vi "Swerve Sensors Read.vi"(11 "Swerve Motor DevRef":T1) -> ()   [LabVIEW 2014]
uses:
  Swerve Sensors DevRef.ctl
  <vilib>/Rock Robotics/WPI/AnalogChannel/WPI_AnalogChannelDevRef.ctl
  <vilib>/Rock Robotics/SystemInterfaces/Typedef/FPGA_TypedefAnalogModule.ctl
  <vilib>/Rock Robotics/SystemInterfaces/AI/FPGA_AIChannel.ctl
  Global Variables/Sensor Data (Edited).vi
  Global Variables/Calibrations.vi
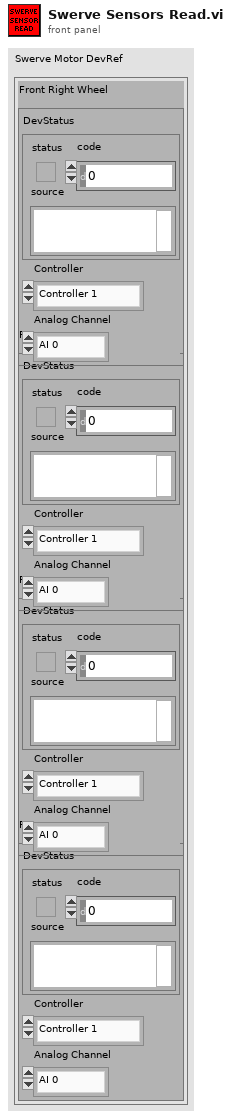
[diagram p1: front panel]
types:
  T1 = typedef "Swerve Sensors DevRef.ctl" = cluster{"Front Right Wheel":T2, "Front Left Wheel":T2, "Rear Right Wheel":T2, "Rear Left Wheel":T2}
  T2 = typedef "WPI_AnalogChannelDevRef.ctl" = cluster{"DevStatus":errorcluster, "Controller":T3, "Analog Channel":T4}
  T3 = typedef "FPGA_TypedefAnalogModule.ctl" = enum16{"Controller 1"}
  T4 = typedef "FPGA_AIChannel.ctl" = enum8{"AI 0", "AI 1", "AI 2", "AI 3", "AI MXP 0", "AI MXP 1", "AI MXP 2", "AI MXP 3", "Invalid"}
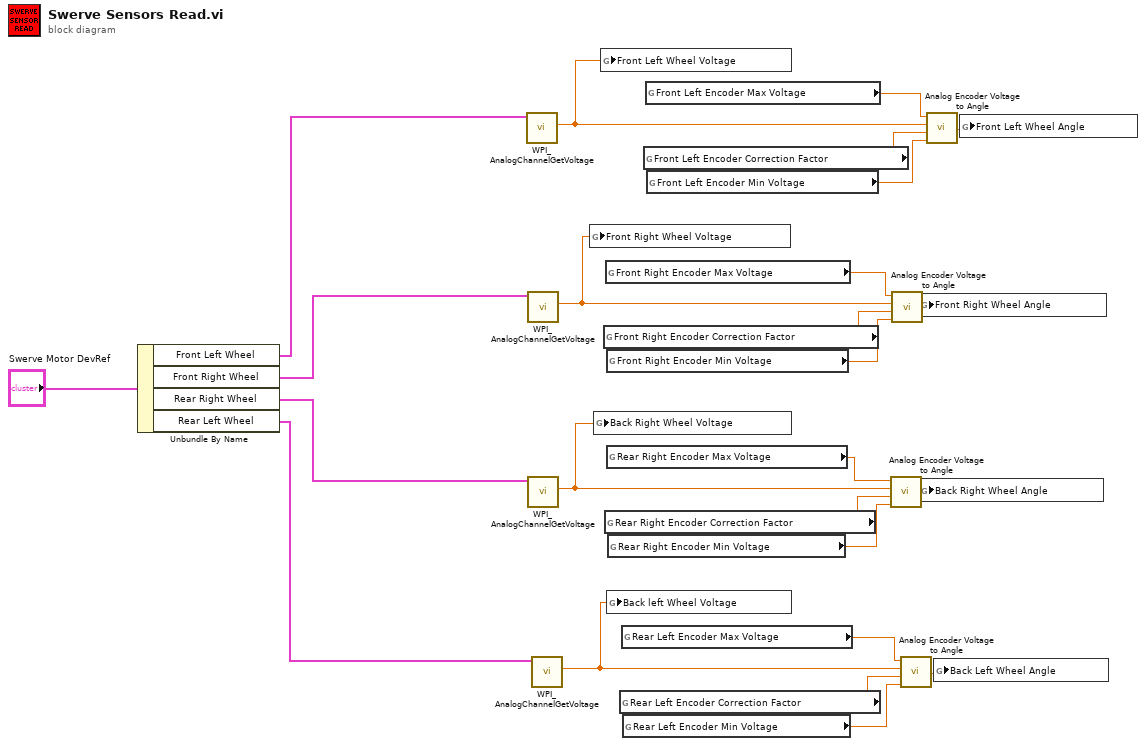
[diagram p0: block diagram]
diagram:
  n1 = Unbundle By Name("Swerve Motor DevRef") -> ("Front Left Wheel"=w24:T2, "Front Right Wheel"=w23:T2, "Rear Right Wheel"=w22:T2, "Rear Left Wheel"=w21:T2)
  n2 = call <vilib>:"WPI_AnalogChannelGetVoltage.vi"("AIDeviceRef"=w24) -> ("Voltage"=w5:dbl)  [unwired: 8 in, 2 out]
  n3 = call <vilib>:"WPI_AnalogChannelGetVoltage.vi"("AIDeviceRef"=w23) -> ("Voltage"=w4:dbl)  [unwired: 8 in, 2 out]
  n4 = call <vilib>:"WPI_AnalogChannelGetVoltage.vi"("AIDeviceRef"=w22) -> ("Voltage"=w2:dbl)  [unwired: 8 in, 2 out]
  n5 = call <vilib>:"WPI_AnalogChannelGetVoltage.vi"("AIDeviceRef"=w21) -> ("Voltage"=w1:dbl)  [unwired: 8 in, 2 out]
  n6 = global write "Sensor Data (Edited).vi" "Front Right Wheel Voltage"(w4) -> ()
  n7 = global write "Sensor Data (Edited).vi" "Back Right Wheel Voltage"(w2) -> ()
  n8 = global write "Sensor Data (Edited).vi" "Front Left Wheel Voltage"(w5) -> ()
  n9 = global read "Calibrations.vi" "Front Right Encoder Correction Factor"() -> (w14:dbl)
  n10 = global read "Calibrations.vi" "Rear Right Encoder Correction Factor"() -> (w11:dbl)
  n11 = global read "Calibrations.vi" "Front Right Encoder Max Voltage"() -> (w15:dbl)
  n12 = global read "Calibrations.vi" "Front Right Encoder Min Voltage"() -> (w13:dbl)
  n13 = global read "Calibrations.vi" "Rear Right Encoder Max Voltage"() -> (w3:dbl)
  n14 = global write "Sensor Data (Edited).vi" "Back left Wheel Voltage"(w1) -> ()
  n15 = global read "Calibrations.vi" "Rear Right Encoder Min Voltage"() -> (w12:dbl)
  n16 = global read "Calibrations.vi" "Rear Left Encoder Correction Factor"() -> (w7:dbl)
  n17 = global read "Calibrations.vi" "Rear Left Encoder Max Voltage"() -> (w8:dbl)
  n18 = global read "Calibrations.vi" "Rear Left Encoder Min Voltage"() -> (w6:dbl)
  n19 = global read "Calibrations.vi" "Front Left Encoder Correction Factor"() -> (w19:dbl)
  n20 = global read "Calibrations.vi" "Front Left Encoder Max Voltage"() -> (w18:dbl)
  n21 = global read "Calibrations.vi" "Front Left Encoder Min Voltage"() -> (w20:dbl)
  n22 = call "Analog Encoder Voltage to Angle.vi"("V-min"=w12, "V-zero"=w11, "Current Votage"=w2, "V-max"=w3) -> ("Angle"=w10:dbl)
  n23 = call "Analog Encoder Voltage to Angle.vi"("V-min"=w13, "V-zero"=w14, "Current Votage"=w4, "V-max"=w15) -> ("Angle"=w16:dbl)
  n24 = call "Analog Encoder Voltage to Angle.vi"("V-min"=w6, "V-zero"=w7, "Current Votage"=w1, "V-max"=w8) -> ("Angle"=w9:dbl)
  n25 = global write "Sensor Data (Edited).vi" "Front Right Wheel Angle"(w16) -> ()
  n26 = global write "Sensor Data (Edited).vi" "Back Right Wheel Angle"(w10) -> ()
  n27 = call "Analog Encoder Voltage to Angle.vi"("V-min"=w20, "V-zero"=w19, "Current Votage"=w5, "V-max"=w18) -> ("Angle"=w17:dbl)
  n28 = global write "Sensor Data (Edited).vi" "Back Left Wheel Angle"(w9) -> ()
  n29 = global write "Sensor Data (Edited).vi" "Front Left Wheel Angle"(w17) -> ()
